vi "S2P IMP Import.vi"(8 "error in (no error)":errorcluster) -> (0 "error out":errorcluster, 3 "Variant Output":variant)   [LabVIEW 2011]
uses:
  TypeDefs/S2P IMP Measurement Data.ctl
  tests/S Parameter/TypeDefs/SP Parameter to Measure.ctl
  tests/S Parameter/TypeDefs/SP Parameter.ctl
  tests/S Parameter/TypeDefs/SP Calibration State.ctl
  tests/S Parameter/TypeDefs/SP Measurement Format.ctl
  tests/S Parameter/TypeDefs/SP Data.ctl
  TypeDefs/S2P IMP Header Info.ctl
panel:
  out "S2P Measurements":T1 {"Parameters Measured"."Channel" min=1 max=99 step=1; "Parameters Measured"."Parameter"."Stimulus Port" min=1 step=1; "Parameters Measured"."Parameter"."Response Port" min=1 step=1}
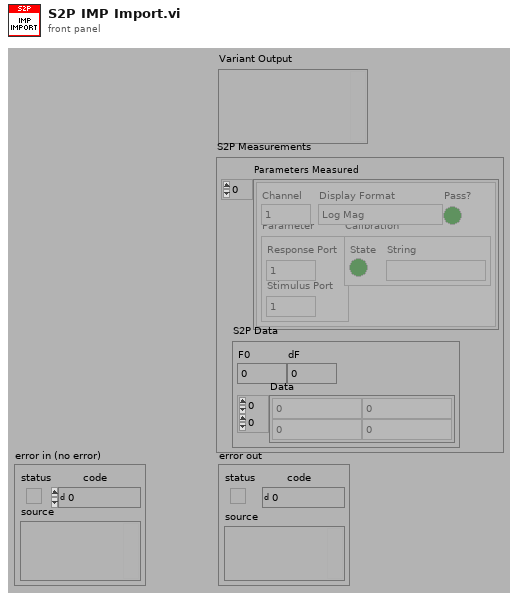
[diagram p1: front panel]
types:
  T1 = typedef "S2P IMP Measurement Data.ctl" = cluster{"Parameters Measured":T2[], "S2P Data":T6}
  T2 = typedef "SP Parameter to Measure.ctl" = cluster{"Channel":i8, "Parameter":T3, "Calibration":T4, "Display Format":T5, "Pass?":bool}
  T3 = typedef "SP Parameter.ctl" = cluster{"Stimulus Port":i8, "Response Port":i8}
  T4 = typedef "SP Calibration State.ctl" = cluster{"State":bool, "String":string}
  T5 = typedef "SP Measurement Format.ctl" = enum32{"Log Mag", "Phase", "Delay", "Smith (R+jX)", "Polar (Re/Im)", "Linear Mag", "SWR", "Real", "Imaginary", "Smith (Lin/Phase)", "Smith (Log/Phase)", "Smith (Real/Imag)", "Smith (G+jB)", "Polar (Lin/Phase)", "Polar (Log/Phase)", "Expanded Phase", "Positive Phase", "Inverted Smith", "Unwrapped Phase", "Power Out", "Power In", "Linear Mag/Phase", "Log Mag/Phase", "Real/Imaginary"}
  T6 = typedef "SP Data.ctl" = cluster{"F0":dbl, "dF":dbl, "Data":cdb[][]}
  T7 = typedef "S2P IMP Header Info.ctl" = cluster{"Frequency Units":string, "Parameter":string, "Format":string, "Reference Resistance":i32}
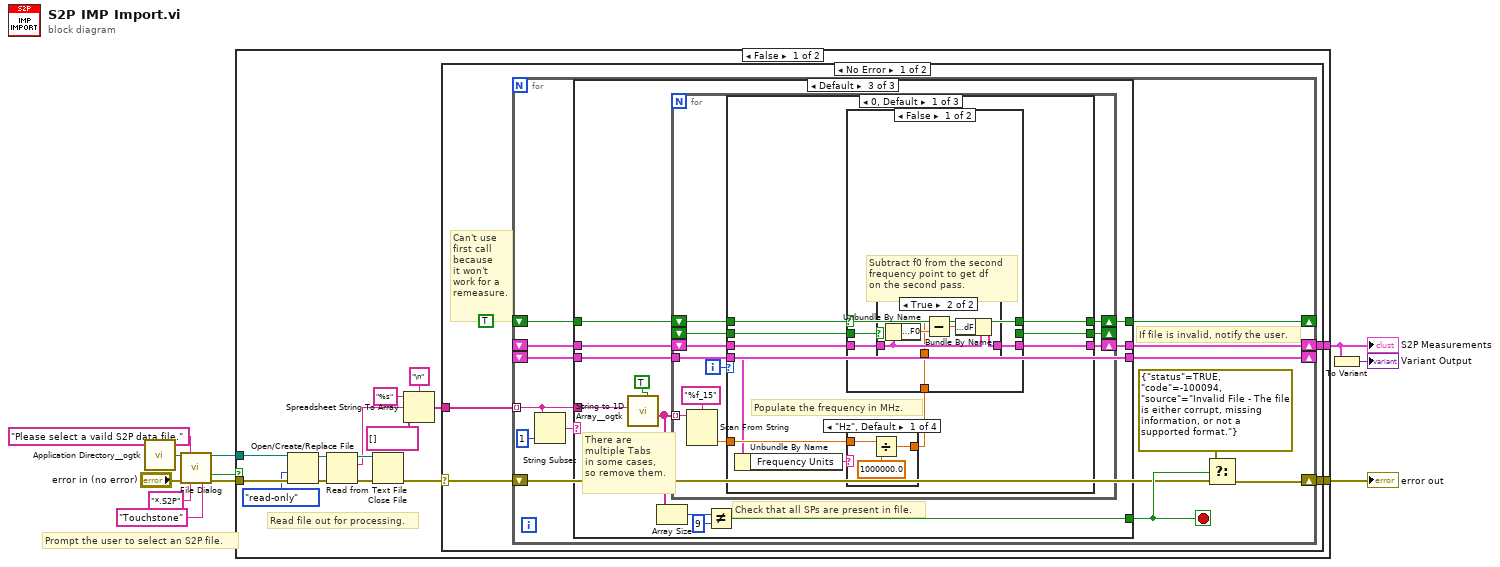
[diagram p0: block diagram]
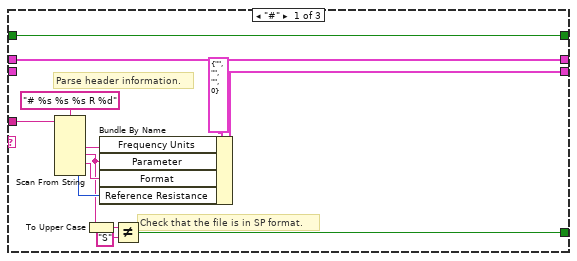
[diagram p2: hidden frame]
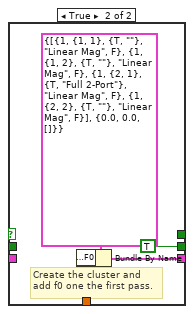
[diagram p5: hidden frame]
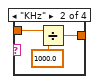
[diagram p6: hidden frame]
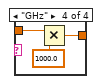
[diagram p8: hidden frame]
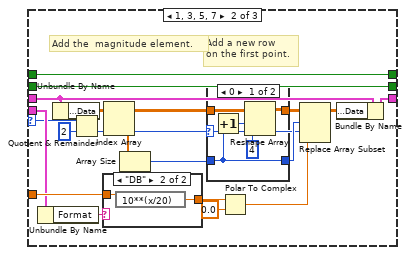
[diagram p9: hidden frame]
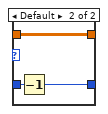
[diagram p10: hidden frame]
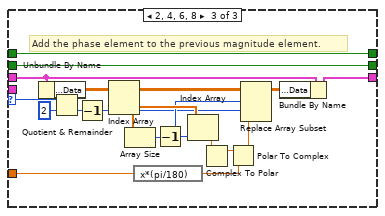
[diagram p12: hidden frame]
diagram:
  # "Prompt the user to select an S2P file."
  n1 = call "Application Directory__ogtk.vi"() -> ("Application Directory (+ Relative)"=w5:path)  [unwired: 1 out]
  n2 = call "File Dialog"("start path"=w5, "prompt"="Please select a vaild S2P data file.", "error in"="error in (no error)", "pattern (all files)"="*.S2P", "pattern label"="Touchstone") -> ("selected path"=w9:path, "cancelled"=w10:bool, "error out"=w11:errorcluster)  [unwired: 2 in, 6 out]
  n3 = case shown="False" w10 {
    tunnel: w11 -> [w26 w167]
    tunnel: w9 -> [w25 _]
    tunnel: [w13 w167] -> w8
    tunnel: [w12 _] -> w7
    frame False {
      # "Read file out for processing."
      n4 = Open/Create/Replace File(file path (use dialog)=w25, error in=w26, access (0:read/write)=enum16{"read/write", "read-only", "write-only"}."read-only") -> (refnum out=w23:refnum<file>, error out=w22:errorcluster)  [unwired: 4 out]
      n5 = Read from Text File(file (use dialog)=w23, error in=w22) -> (refnum out=w20:refnum<file>, text=w19:string, error out=w21:errorcluster)  [unwired: 3 out]
      n6 = Close File(refnum=w20, error in=w21) -> (error out=w14:errorcluster)  [unwired: 1 out]
      n7 = Spreadsheet String To Array(delimiter (Tab)="\n", format string="%s", spreadsheet string=w19, array type (2D Dbl)=string[] []) -> (array=w15:string[])
      n8 = case shown="No Error" w14 {
        selector: w14 -> [w30 w166]
        tunnel: w15 -> [w31 _]
        tunnel: [w29 w166] -> w13
        tunnel: [w28 _] -> w12
        frame No Error {
          # "Can't use\nfirst call\nbecause\nit won't\nwork for a\nremeasure."
          n9 = for {
            tunnel: w31 -> [w40] mode=indexing
            shift-right: [w44] -> _
            shift-left: _ -> [w43]
            shift-right: [w37] -> w29
            shift-left: w30 -> [w38]
            shift-right: [w35] -> w28
            shift-left: _ -> [w34]
            shift-right: [w32] -> _
            shift-left: TRUE ("ignore duplicate delimiters? (F=No)") -> [w33]
            stop <- w39 stop-if-true
            # "If file is invalid, notify the user."
            n10 = String Subset(string=w40, length (rest)=1 ("length (rest)")) -> (substring=w41:string)  [unwired: 1 out]
            n11 = case shown="Default" w41 {
              tunnel: [w52 w60 w71] -> w44
              tunnel: w43 -> [_ w60 w71]
              tunnel: w40 -> [w51 _ w66]
              tunnel: [w47 _ w64] -> w39
              tunnel: [w46 w59 w68] -> w35
              tunnel: w34 -> [w46 w59 w67]
              tunnel: w33 -> [w45 w58 w62]
              tunnel: [w45 w58 w61] -> w32
              frame "#" {
                # "Check that the file is in SP format."
                # "Parse header information."
                n12 = Scan From String(format string="# %s %s %s R %d", input string=w51) -> (output 1=w55:string, output 2=w50:string, output 3=w54:string, output 4=w53:i32)  [unwired: 2 in, 7 out]
                n13 = To Upper Case(1:w50) -> (0:w49:string)
                n14 = Bundle By Name(cluster=T7 {"Frequency Units"="", "Parameter"="", "Format"="", "Reference Resistance"=0} ("S2P Header Info"), "Frequency Units"=w55, "Parameter"=w50, "Format"=w54, "Reference Resistance"=w53) -> (w52:T7)
                n15 = Not Equal?(x=w49, y="S") -> (x != y?=w47:bool)
              }
              frame "", "!" {
                # "Ignore any comment or blank lines."
              }
              frame Default {
                # "Check that all SPs are present in file."
                # "There are\nmultiple Tabs\nin some cases,\nso remove them."
                n16 = call "String to 1D Array__ogtk.vi"("ignore duplicate delimiters? (F=No)"=TRUE, "string"=w66) -> ("Array of Strings"=w63:string[])  [unwired: 1 in, 8 out]
                n17 = Array Size(array=w63) -> (size(s)=w70:i32)
                n18 = for {
                  tunnel: w71 -> [w81]
                  tunnel: w63 -> [w77] mode=indexing
                  shift-right: [w80] -> w68
                  shift-left: w67 -> [w79]
                  shift-right: [w72] -> w61
                  shift-left: w62 -> [w75]
                  shift-right: [w73] -> _
                  shift-left: _ -> [w74]
                  i -> [w82]
                  n19 = Scan From String(format string="%f_15", input string=w77) -> (output 1=w78:dbl)  [unwired: 2 in, 4 out]
                  n20 = case shown="0, Default" w82 {
                    selector: w82 -> [_ w133 w160]
                    tunnel: w78 -> [w91 w135 w156]
                    tunnel: w81 -> [w90 w134 _]
                    tunnel: [w88 w129 w162] -> w80
                    tunnel: w79 -> [w87 w130 w163]
                    tunnel: w75 -> [w86 w118 w148]
                    tunnel: w74 -> [w85 w119 w149]
                    tunnel: [w84 w119 w149] -> w73
                    tunnel: [w83 w118 w148] -> w72
                    frame 0, Default {
                      # "Populate the frequency in MHz."
                      n21 = Unbundle By Name(w90) -> ("Frequency Units"=w92:string)
                      n22 = case shown="\"Hz\", Default" w92 {
                        tunnel: w91 -> [w110 w113 w114 w117]
                        tunnel: [w108 w111 w114 w115] -> w89
                        frame "Hz", Default {
                          n23 = Divide(x=w110, y=1000000.0) -> (x/y=w108:dbl)
                        }
                        frame "KHz" {
                          n24 = Divide(x=w113, y=1000.0) -> (x/y=w111:dbl)
                        }
                        frame "MHz" {
                        }
                        frame "GHz" {
                          n25 = Multiply(x=w117, y=1000.0) -> (x*y=w115:dbl)
                        }
                      }
                      n26 = case shown="False" w86 {
                        selector: w86 -> [w93 _]
                        tunnel: w89 -> [w95 w105]
                        tunnel: [w96 w106] -> w88
                        tunnel: w87 -> [w97 _]
                        tunnel: w85 -> [w94 _]
                        tunnel: [_ TRUE ("ignore duplicate delimiters? (F=No)")] -> w84
                        tunnel: [w93 _] -> w83
                        frame False {
                          # "Subtract f0 from the second\nfrequency point to get df\non the second pass."
                          n27 = case shown="True" w94 {
                            tunnel: w97 -> [w98 w102]
                            tunnel: [w98 w103] -> w96
                            tunnel: w95 -> [_ w99]
                            frame False {
                            }
                            frame True {
                              n28 = Unbundle By Name(w102) -> ("S2P Data.F0"=w101:dbl)
                              n29 = Subtract(x=w99, y=w101) -> (x-y=w100:dbl)
                              n30 = Bundle By Name(cluster=w102, "S2P Data.dF"=w100) -> (w103:T1)
                            }
                          }
                        }
                        frame True {
                          # "Create the cluster and\nadd f0 one the first pass."
                          n31 = Bundle By Name(cluster=T1 {"Parameters Measured"=[{"Channel"=1, "Parameter"={"Stimulus Port"=1, "Response Port"=1}, "Calibration"={"State"=TRUE, "String"=""}, "Display Format"=enum."Linear Mag", "Pass?"=FALSE}, {"Channel"=1, "Parameter"={"Stimulus Port"=1, "Response Port"=2}, "Calibration"={"State"=TRUE, "String"=""}, "Display Format"=enum."Linear Mag", "Pass?"=FALSE}, {"Channel"=1, "Parameter"={"Stimulus Port"=2, "Response Port"=1}, "Calibration"={"State"=TRUE, "String"="Full 2-Port"}, "Display Format"=enum."Linear Mag", "Pass?"=FALSE}, {"Channel"=1, "Parameter"={"Stimulus Port"=2, "Response Port"=2}, "Calibration"={"State"=TRUE, "String"=""}, "Display Format"=enum."Linear Mag", "Pass?"=FALSE}], "S2P Data"={"F0"=0.0, "dF"=0.0, "Data"=[]}} ("S2P Measurements"), "S2P Data.F0"=w105) -> (w106:T1)
                        }
                      }
                    }
                    frame 1, 3, 5, 7 {
                      # "Add the  magnitude element."
                      # "Add a new row\non the first point."
                      n32 = Unbundle By Name(w134) -> ("Format"=w136:string)
                      n33 = Unbundle By Name(w130) -> ("S2P Data.Data"=w128:cdb[][])
                      n34 = Quotient & Remainder(x=w133, y=2) -> (floor(x/y)=w120:i32)  [unwired: 1 out]
                      n35 = case shown="\"DB\"" w136 {
                        tunnel: w135 -> [w145 w147]
                        tunnel: [w145 w146] -> w131
                        frame "MA", "RI", Default {
                        }
                        frame "DB" {
                          n36 = expression code="10**(x/20)"(w147) -> (w146:dbl)
                        }
                      }
                      n37 = Index Array(array=w128, index (col)=w120) -> (element=w124:cdb[])  [unwired: 1 in]
                      n38 = Array Size(array=w124) -> (size(s)=w122:i32)
                      n39 = case shown="0" w120 {
                        tunnel: w128 -> [w141 w144]
                        tunnel: [w140 w144] -> w125
                        tunnel: w122 -> [w137 w143]
                        tunnel: [w137 w142] -> w121
                        frame 0 {
                          n40 = Increment(x=w137) -> (x+1=w138:i32)
                          n41 = Reshape Array(w141, w138, 4 ("dimension size")) -> (w140:cdb[][])
                        }
                        frame Default {
                          n42 = Decrement(x=w143) -> (x-1=w142:i32)
                        }
                      }
                      n43 = Polar To Complex(1:0.0 ("theta"), 2:w131) -> (0:w123:cdb)
                      n44 = Replace Array Subset(array=w125, new element=w123, index (row)=w121, index (col)=w120) -> (w127:cdb[][])
                      n45 = Bundle By Name(cluster=w130, "S2P Data.Data"=w127) -> (w129:T1)
                    }
                    frame 2, 4, 6, 8 {
                      # "Add the phase element to the previous magnitude element."
                      n46 = Unbundle By Name(w163) -> ("S2P Data.Data"=w161:cdb[][])
                      n47 = Quotient & Remainder(x=w160, y=2) -> (floor(x/y)=w154:i32)  [unwired: 1 out]
                      n48 = Decrement(x=w154) -> (x-1=w150:i32)
                      n49 = Index Array(array=w161, index (col)=w150) -> (element=w157:cdb[])  [unwired: 1 in]
                      n50 = Array Size(array=w157) -> (size(s)=w153:i32)
                      n51 = expression code="x*(pi/180)"(w156) -> (w155:dbl)
                      n52 = Decrement(x=w153) -> (x-1=w152:i32)
                      n53 = Index Array(array=w157, index=w152) -> (element=w159:cdb)
                      n54 = Complex To Polar(r * e^(i*theta)=w159) -> (r=w158:dbl)  [unwired: 1 out]
                      n55 = Polar To Complex(1:w155, 2:w158) -> (0:w151:cdb)
                      n56 = Replace Array Subset(array=w161, new element=w151, index (row)=w152, index (col)=w150) -> (w164:cdb[][])
                      n57 = Bundle By Name(cluster=w163, "S2P Data.Data"=w164) -> (w162:T1)
                    }
                  }
                }
                n58 = Not Equal?(x=w70, y=9) -> (x != y?=w64:bool)
              }
            }
            n59 = Select(t=errorcluster {"status"=TRUE, "code"=-100094, "source"="Invalid File - The file is either corrupt, missing information, or not a supported format."}, s=w39, f=w38) -> (s? t:f=w37:errorcluster)
          }
        }
        frame Error {
        }
      }
    }
    frame True {
    }
  }
  "error out" <- w8
  "S2P Measurements" <- w7
  n60 = To Variant(anything=w7) -> (Variant=→"Variant Output":variant)
